vi "main_locate.vi"() -> ()   [LabVIEW 2023]
uses:
  subVis/HologramInfo.ctl
  <vilib>/Math Plots/3D Math Plots/3D Scatter/3D Scatter XCtrl/3D Scatter.xctl
  <vilib>/Math Plots/3D Math Plots/3D Scatter/3D Scatter Datatype/3D Scatter Datatype.lvclass
  HoloPyLib/CCL_parameters.ctl
  subVis/referencesBtns.ctl
  subVis/datas.ctl
  <vilib>/Math Plots/3D Math Plots/3D Scatter/3D Scatter Datatype/Public/Plot Helper (Vector).vi
  subVis/globState.vi
  <vilib>/Python/Open Venv Python Session.vi
  HoloPyLib/holoPyTracks.lvlib
panel:
  out "Status":string
  in  "result tab":enum32{"Holograms", "Localisations", "About..."}(tab)
  out "2D Picture":picture caption="Hologram plane number 152"
  out "3D Scatter":refnum<class "3D Plot Datatype.lvclass">[](xcontrol)
  in  "Tab Control":enum32{"PATH", "PARAMETERS", "ACTIONS"}(tab)=enum."ACTIONS"
  in  "HoloDir":path=path "C:/TRAVAIL/developpement/imagesHolo/1000im_manip3" caption="Holograms directory"
  in  "HoloPath":path=path "C:/TRAVAIL/developpement/imagesHolo/1000im_manip3/100um_40x_int_.7ajmvz4e.000000.bmp" caption="Test hologram path"
  in  "PythonVer":string="3.10" caption="Python version"
  in  "Python/Environnement\npath":path
  in  "Fourier BP filter (pix)":T1={"High pass (0=none)"=15.0, "Low Pass (0=none)"=125.0} {"Low Pass (0=none)" format="%#_6f"}
  in  "CCL parameters":T2={"Threshold ( N x Standard deviation)"=10.0, "Connectivity"=enum."26", "min voxel"=1.0, "max voxel"=0.0} {"max voxel" min=0.0 max=0.0; "min voxel" min=1.0 max=100.0; "Threshold ( N x Standard deviation)" min=1.0 max=100.0}
  in  "Batch thresold":T3(ring)
  in  "Focus":T4={"Type"=enum."SUM_OF_VARIANCE", "Sum size"=15} {"Sum size" min=1 max=100}
  in  "propagation":T5={"distance ini"=0.0, "number of planes"=100, "step"=1e-06} {"step" format="%#_6e"; "distance ini" format="%#_6e"}
  in  "Remove mean Hologram":bool=TRUE
  in  "HoloParam":T6={"wavelength"=6.6e-07, "optical index"=1.33, "Holo size X"=1024, "Holo size Y"=1024, "pixel size"=7e-06, "objective magnification"=40.0} caption="Holo parameters" {"wavelength" format="%#_6e"}
  in  "exitTestMode":bool
  in  "testMode":bool
  in  "CANCEL_BATCH":bool
  in  "EXIT":bool
  in  "BATCH":bool
  in  "Plane number":u16=95 max=200
  in  "Display":T7(ring)
  # "Analyse parameters"
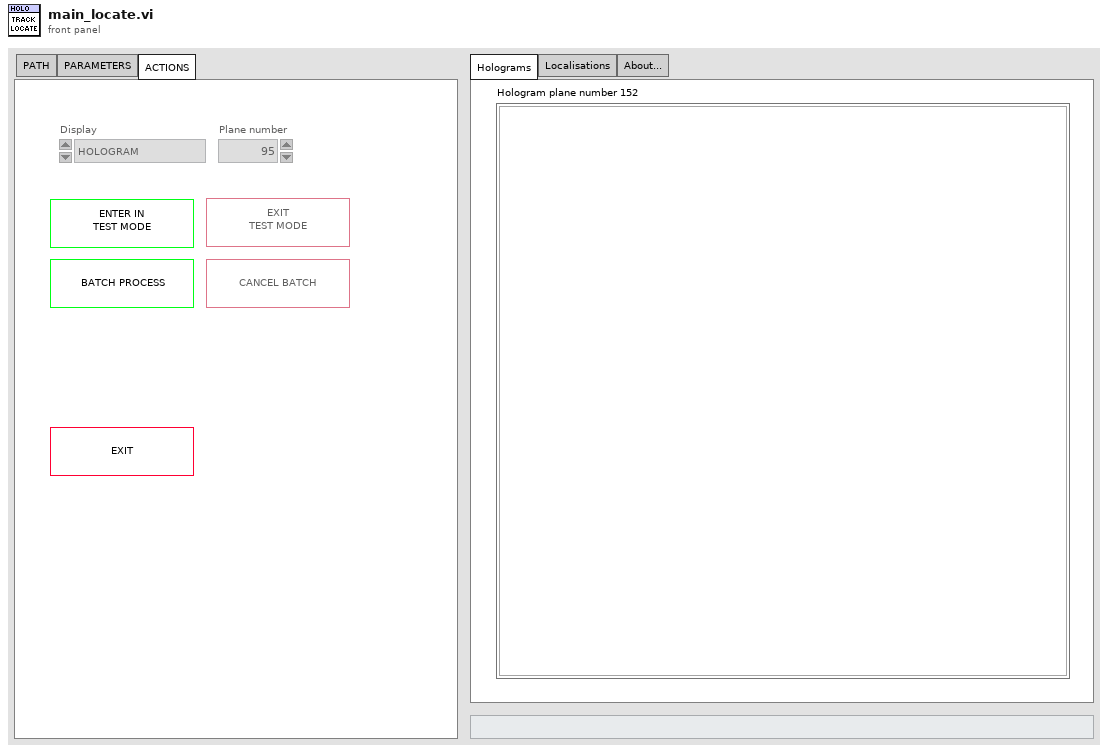
[diagram p1: front panel]
types:
  T1 = cluster{"High pass (0=none)":dbl, "Low Pass (0=none)":dbl}
  T2 = typedef "CCL_parameters.ctl" = cluster{"Threshold ( N x Standard deviation)":dbl, "Connectivity":enum16{"6", "18", "26"}, "min voxel":dbl, "max voxel":dbl}
  T3 = enum16{"compute on 1st hologram", "compute on each hologram"}
  T4 = cluster{"Type":enum16{"SUM_OF_INTENSITY", "SUM_OF_LAPLACIAN", "SUM_OF_VARIANCE", "TENENGRAD"}, "Sum size":i32}
  T5 = cluster{"distance ini":dbl, "number of planes":i32, "step":dbl}
  T6 = typedef "holoPyTracks.lvlib/HologramInfo.ctl" = cluster{"wavelength":sgl, "optical index":sgl, "Holo size X":i32, "Holo size Y":i32, "pixel size":sgl, "objective magnification":sgl}
  T7 = enum16{"HOLOGRAM", "XY PLANE NUMBER....", "XY MAX PLANE", "XY SUM PLANE", "XZ MAX PLANE", "XZ SUM PLANE", "YZ MAX PLANE", "YZ SUM PLANE"}
  T8 = typedef "referencesBtns.ctl" = cluster{"PythonVer":refnum<vi>, "Python/Environnement\npath":refnum<vi>, "HoloPath":refnum<vi>, "HoloDir":refnum<vi>, "Holo parameters":refnum<vi>, "Remove mean Hologram":refnum<vi>, "propagation":refnum<vi>, "Fourier BP filter (pix)":refnum<vi>, "Focus":refnum<vi>, "Batch thresold ":refnum<vi>, "CCL parameters":refnum<vi>, "testMode":refnum<vi>, "exitTestMode":refnum<vi>, "BATCH":refnum<vi>, "CANCEL_BATCH":refnum<vi>, "EXIT":refnum<vi>, "Plane number":refnum<vi>, "Display":refnum<vi>}
  T9 = typedef "param_defaut.ctl" = cluster{"PythonVer":string, "Python/Environnement\npath":path, "HoloPath":path, "HoloDir":path, "HoloParam":T6, "Remove mean Hologram":bool, "propagation":cluster{"distance ini":dbl, "number of planes":i32, "step":dbl}, "Fourier BP filter (pix)":cluster{"High pass (0=none)":dbl, "Low Pass (0=none)":dbl}, "Focus":cluster{"Type":enum16{"SUM_OF_INTENSITY", "SUM_OF_LAPLACIAN", "SUM_OF_VARIANCE", "TENENGRAD"}, "Sum size":i32}, "Batch thresold ":enum16{"compute on 1st hologram", "compute on each hologram"}, "CCL parameters":T2}
  T10 = enum16{"SESSION CLOSED", "WAIT", "TEST WAIT", "TEST IN PROGESS", "BATCH IN PROGRESS"}
  T11 = typedef "datas.ctl" = cluster{"PythonSession":refnum<k35>, "Display":bool, "BinThreshold":sgl, "LIST HOLO BATCH":path[], "Display":sgl[][], "meanHolo":sgl[][], "FEATURES(µm)":sgl[][], "LabelPicture":string, "Status":string, "planeToDisplayFeatures":enum16{"XY", "XZ", "YZ"}, "State":enum16{"SESSION CLOSED", "WAIT", "TEST WAIT", "TEST IN PROGESS", "BATCH IN PROGRESS"}}
  T12 = cluster{"Remove mean Hologram":bool, "Binarisation thresold ":enum16{"compute on 1st hologram", "compute on each hologram"}, "LIST HOLO BATCH":path[], "HoloDir":path}
  T13 = cluster{"Holo parameters":T6, "propagation":cluster{"distance ini":dbl, "number of planes":i32, "step":dbl}, "Fourier BP filter (pix)":cluster{"High pass (0=none)":dbl, "Low Pass (0=none)":dbl}, "Focus":cluster{"Type":enum16{"SUM_OF_INTENSITY", "SUM_OF_LAPLACIAN", "SUM_OF_VARIANCE", "TENENGRAD"}, "Sum size":i32}, "CCL parameters":T2}
  T14 = cluster{"Display":enum16{"HOLOGRAM", "XY PLANE NUMBER....", "XY MAX PLANE", "XY SUM PLANE", "XZ MAX PLANE", "XZ SUM PLANE", "YZ MAX PLANE", "YZ SUM PLANE"}, "Plane number":u16}
  T15 = cluster{"HOLO_array":sgl[][], "FEATURES(µm)":sgl[][], "Features(pix)":sgl[][], "planeToDisplayFeatures":enum16{"XY", "XZ", "YZ"}, "label":string}
  T16 = cluster{"X":i32, "Y":i32, "Z":i32, "XYsize":i32, "ZSize":i32}
  T17 = typedef "eventvkey.ctl" = enum16{"ASCII", "Enter", "Return", "Shift", "Ctrl", "Alt", "Cmd", "Opt", "Caps", "NumLock", "Clear", "Break", "Up", "Down", "Left", "Right", "Insert", "Delete", "Home", "End", "PageUp", "PageDown", "Escape", "Help", "Pause", "ScrollLock", "F1", "F2", "F3", "F4", "F5", "F6", "F7", "F8", "F9", "F10", "F11", "F12", "F13", "F14", "F15", "F16", "F17", "F18", "F19", "F20", "F21", "F22", "F23", "F24", "Play", "VolumeUp", "VolumeDown", "Mute", "Two Byte Char"}
  T18 = cluster{"Display":enum16{"HOLOGRAM", "XY PLANE NUMBER....", "XY MAX PLANE", "XY SUM PLANE", "XZ MAX PLANE", "XZ SUM PLANE", "YZ MAX PLANE", "YZ SUM PLANE"}, u16}
  T19 = cluster{"PythonVer":string, "Python/Environnement\npath":path, "HoloPath":path, "HoloDir":path, "HoloParam":T6, "Remove mean Hologram":bool, "propagation":cluster{"distance ini":dbl, "number of planes":i32, "step":dbl}, "Fourier BP filter (pix)":cluster{"High pass (0=none)":dbl, "Low Pass (0=none)":dbl}, "Focus":cluster{"Type":enum16{"SUM_OF_INTENSITY", "SUM_OF_LAPLACIAN", "SUM_OF_VARIANCE", "TENENGRAD"}, "Sum size":i32}, "Batch thresold ":enum16{"compute on 1st hologram", "compute on each hologram"}, "CCL parameters":T2}
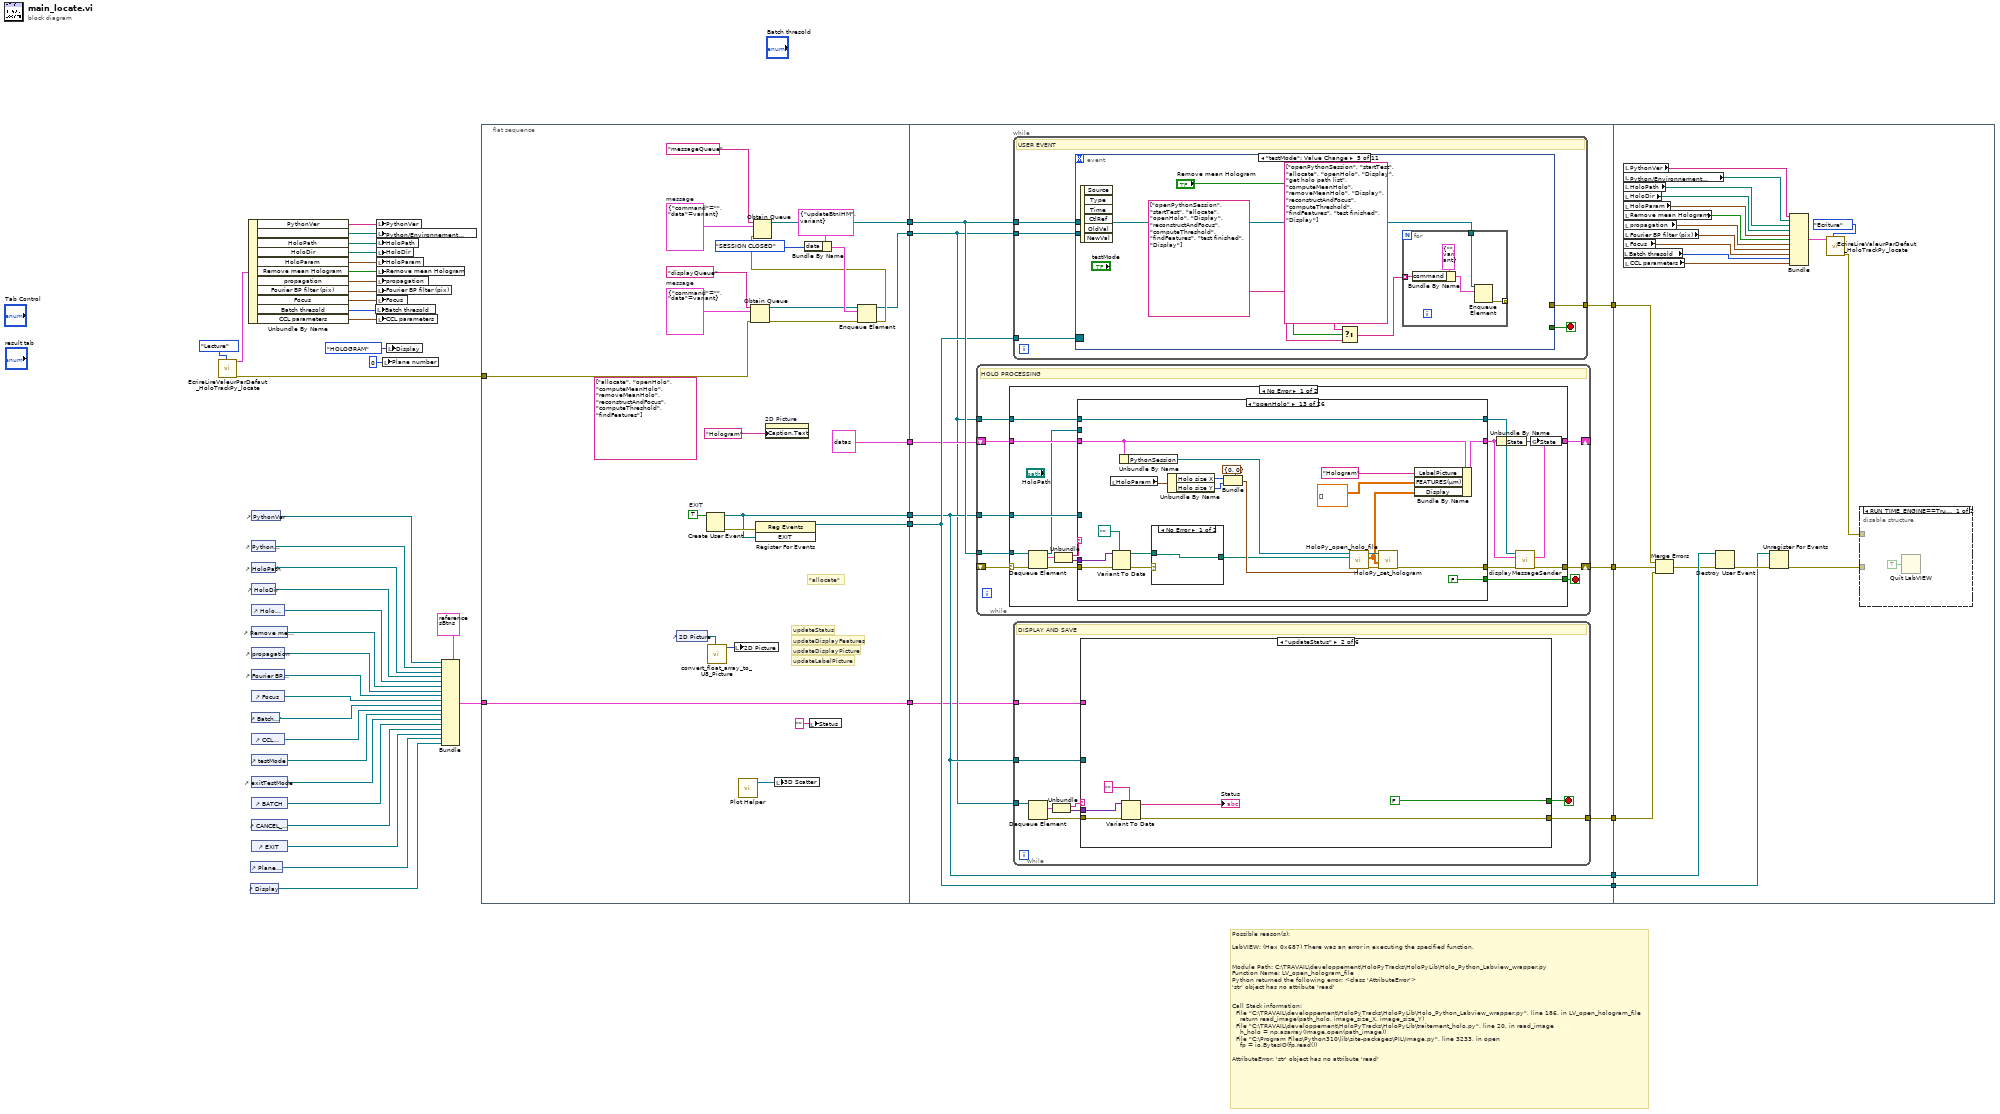
[diagram p0: block diagram]
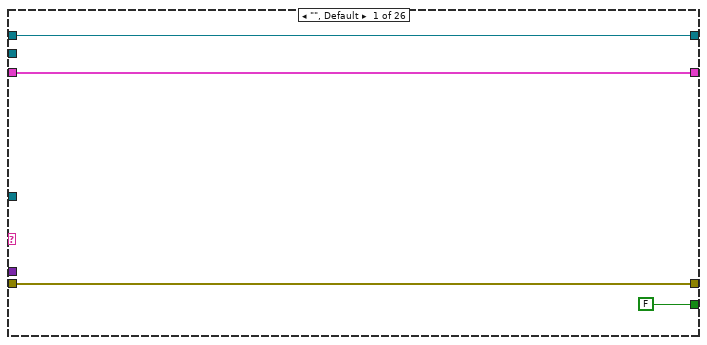
[diagram p2: hidden frame]
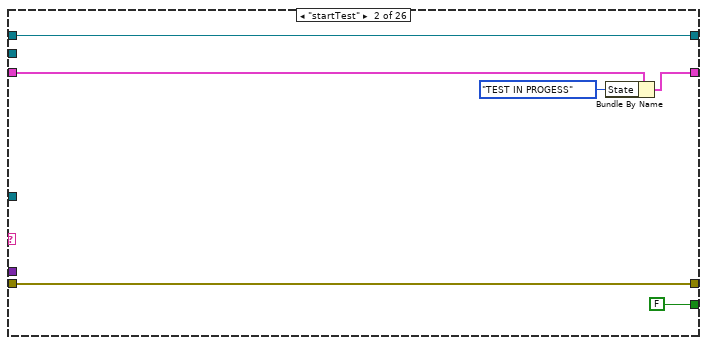
[diagram p3: hidden frame]
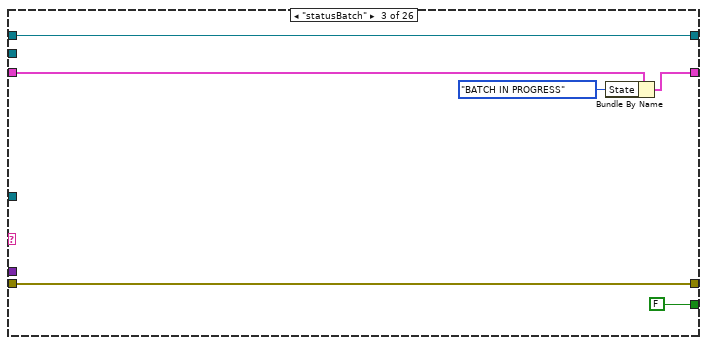
[diagram p4: hidden frame]
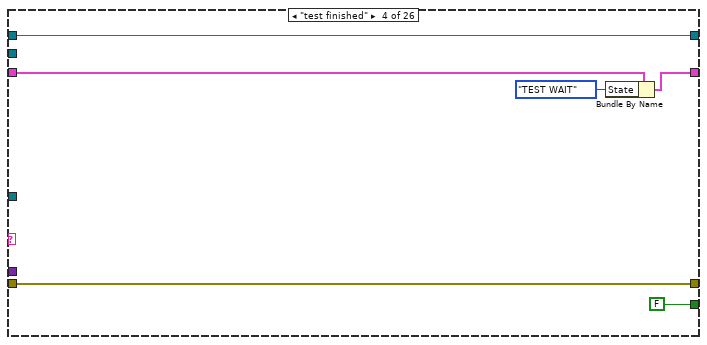
[diagram p5: hidden frame]
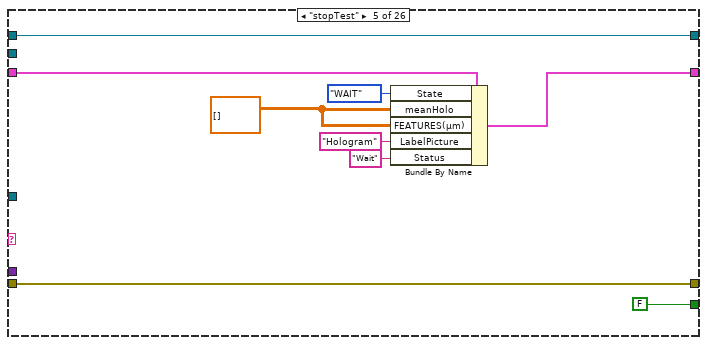
[diagram p6: hidden frame]
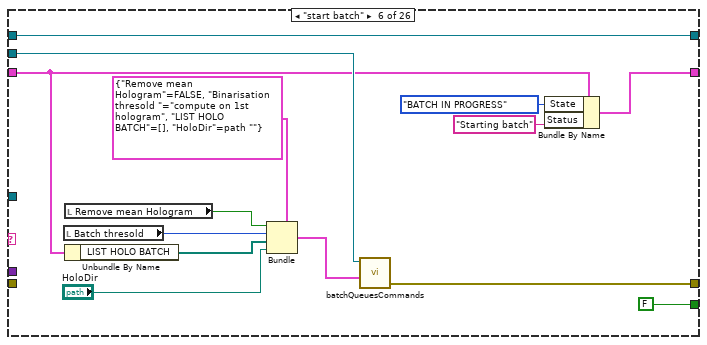
[diagram p7: hidden frame]
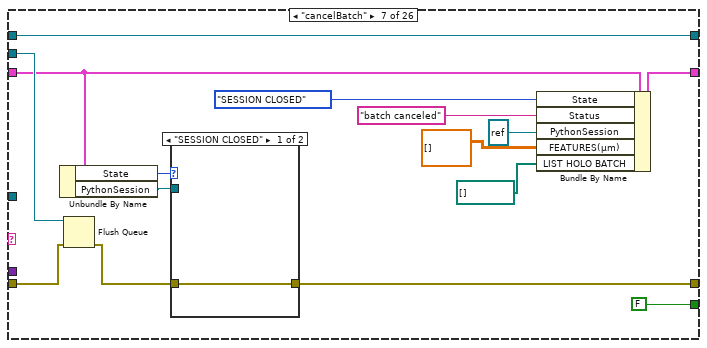
[diagram p8: hidden frame]
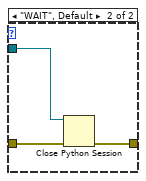
[diagram p9: hidden frame]
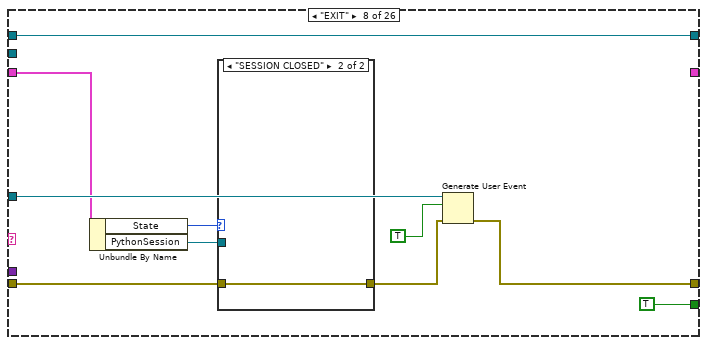
[diagram p10: hidden frame]
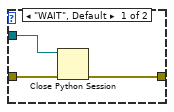
[diagram p11: hidden frame]
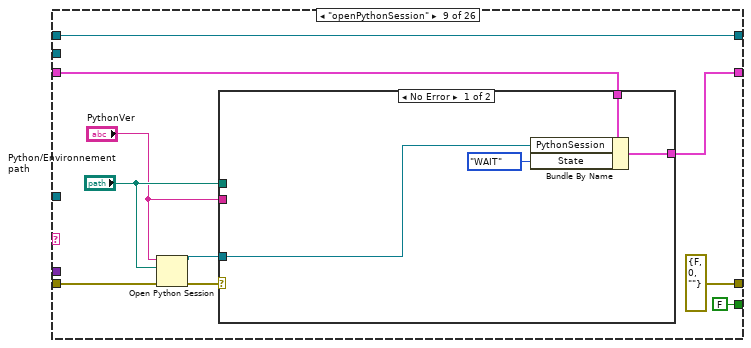
[diagram p12: hidden frame]
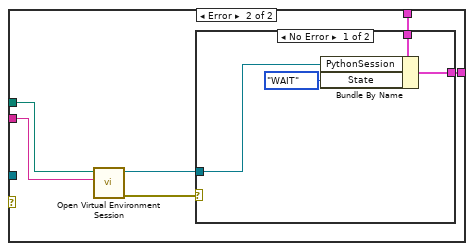
[diagram p13: hidden frame]
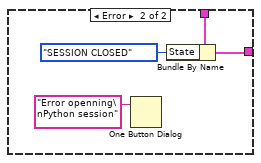
[diagram p14: hidden frame]
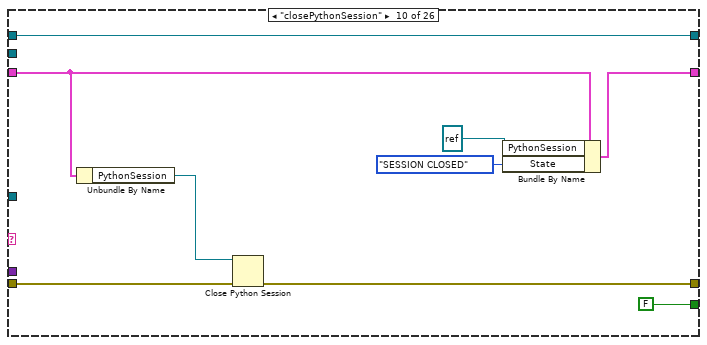
[diagram p15: hidden frame]
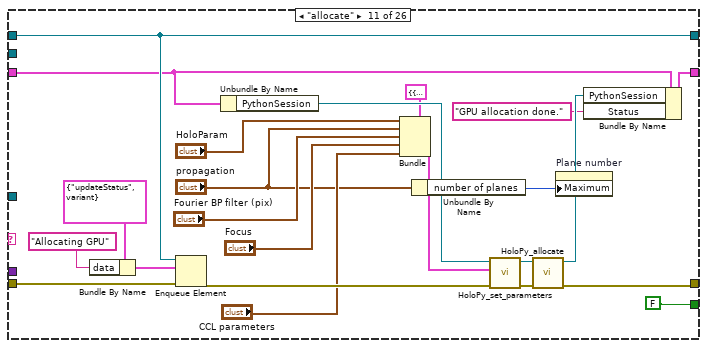
[diagram p16: hidden frame]
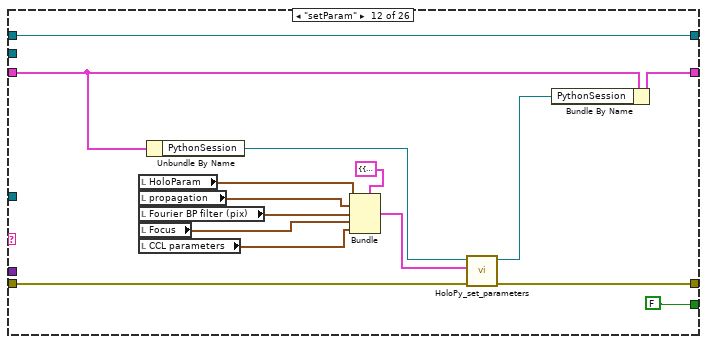
[diagram p17: hidden frame]
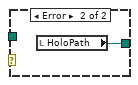
[diagram p18: hidden frame]
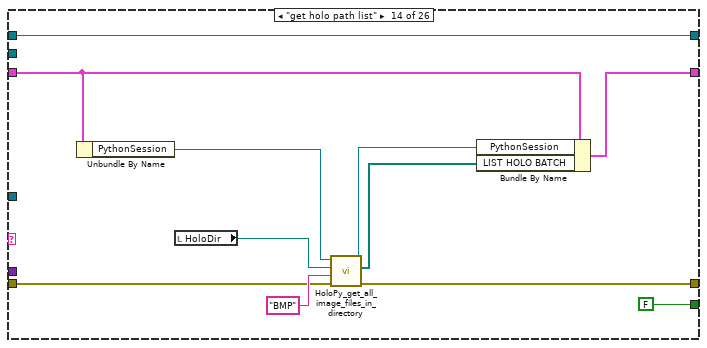
[diagram p19: hidden frame]
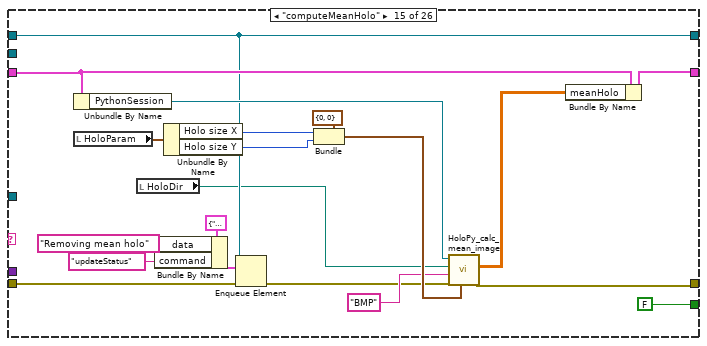
[diagram p20: hidden frame]
diagram:
  # "Possible reason(s):\n\nLabVIEW: (Hex 0x687) There was an error in executing the specified function.\n\n\nModule Path: C:\\TRAVAIL\\developpement\\HoloPyTracks\\HoloPyLib\\Holo_Python_Labview_wrapper.py\nFunction Name: LV_open_hologram_file\nPython returned the following error: <class 'AttributeError'>\n'str' object has no attribute 'read'\n\n\nCall Stack information:\n  File \"C:\\TRAVAIL\\developpement\\HoloPyTracks\\HoloPyLib\\Holo_Python_Labview_wrapper.py\", line 186, in LV_open_hologram_file\n    return read_image(path_holo, image_size_X, image_size_Y)\n  File \"C:\\TRAVAIL\\developpement\\HoloPyTracks\\HoloPyLib\\traitement_holo.py\", line 20, in read_image\n    h_holo = np.asarray(Image.open(path_image))\n  File \"C:\\Program Files\\Python310\\lib\\site-packages\\PIL\\Image.py\", line 3233, in open\n    fp = io.BytesIO(fp.read())\n\nAttributeError: 'str' object has no attribute 'read'"
  n1 = call "EcrireLireValeurParDefaut_HoloTrackPy_locate.vi"("Lecture/Ecriture"=enum32{"Lecture", "Ecriture"}."Lecture") -> ("error out"=w31:errorcluster, "ParamOUT"=w33:T9)  [unwired: 7 in, 2 out]
  n2 = Unbundle By Name(w33) -> ("PythonVer"=w18:string, "Python/Environnement\npath"=w17:path, "HoloPath"=w16:path, "HoloDir"=w15:path, "HoloParam"=w14:T6, "Remove mean Hologram"=w13:bool, "propagation"=w12:T5, "Fourier BP filter (pix)"=w11:T1, "Focus"=w10:T4, "Batch thresold"=w9:T3, "CCL parameters"=w8:T2)
  n3 = control-ref of="Plane number"() -> (w7:refnum<vi>)
  n4 = control-ref of="Display"() -> (w1:refnum<vi>)
  n5 = control-ref of="PythonVer"() -> (w29:refnum<vi>)
  n6 = control-ref of="Python/Environnement\npath"() -> (w30:refnum<vi>)
  n7 = control-ref of="HoloPath"() -> (w38:refnum<vi>)
  n8 = control-ref of="HoloDir"() -> (w37:refnum<vi>)
  n9 = control-ref of="Holo parameters"() -> (w36:refnum<vi>)
  n10 = control-ref of="Remove mean Hologram"() -> (w28:refnum<vi>)
  n11 = control-ref of="propagation"() -> (w27:refnum<vi>)
  n12 = control-ref of="Fourier BP filter (pix)"() -> (w26:refnum<vi>)
  n13 = control-ref of="Focus"() -> (w25:refnum<vi>)
  n14 = control-ref of="Batch thresold"() -> (w24:refnum<vi>)
  n15 = control-ref of="CCL parameters"() -> (w23:refnum<vi>)
  n16 = control-ref of="testMode"() -> (w22:refnum<vi>)
  n17 = control-ref of="exitTestMode"() -> (w21:refnum<vi>)
  n18 = control-ref of="BATCH"() -> (w20:refnum<vi>)
  n19 = control-ref of="CANCEL_BATCH"() -> (w19:refnum<vi>)
  n20 = control-ref of="EXIT"() -> (w35:refnum<vi>)
  n21 = local write "Batch thresold"(w9) -> ()
  n22 = local write "PythonVer"(w18) -> ()
  n23 = local write "Python/Environnement\npath"(w17) -> ()
  n24 = local write "HoloPath"(w16) -> ()
  n25 = local write "HoloDir"(w15) -> ()
  n26 = local write "HoloParam"(w14) -> ()
  n27 = local write "Remove mean Hologram"(w13) -> ()
  n28 = local write "propagation"(w12) -> ()
  n29 = local write "Fourier BP filter (pix)"(w11) -> ()
  n30 = local write "Focus"(w10) -> ()
  n31 = local write "CCL parameters"(w8) -> ()
  n32 = local write "Plane number"(u16 0 ("Plane number")) -> ()
  n33 = local write "Display"(T7."HOLOGRAM" ("Display")) -> ()
  n34 = Bundle(cluster=T8 {"PythonVer"=refnum, "Python/Environnement\npath"=refnum, "HoloPath"=refnum, "HoloDir"=refnum, "Holo parameters"=refnum, "Remove mean Hologram"=refnum, "propagation"=refnum, "Fourier BP filter (pix)"=refnum, "Focus"=refnum, "Batch thresold "=refnum, "CCL parameters"=refnum, "testMode"=refnum, "exitTestMode"=refnum, "BATCH"=refnum, "CANCEL_BATCH"=refnum, "EXIT"=refnum, "Plane number"=refnum, "Display"=refnum} ("output cluster"), "PythonVer"=w29, "Python/Environnement\npath"=w30, "HoloPath"=w38, "HoloDir"=w37, "Holo parameters"=w36, "Remove mean Hologram"=w28, "propagation"=w27, "Fourier BP filter (pix)"=w26, "Focus"=w25, "Batch thresold"=w24, "CCL parameters"=w23, "testMode"=w22, "exitTestMode"=w21, "BATCH"=w20, "CANCEL_BATCH"=w19, "EXIT"=w35, "Plane number"=w7, "Display"=w1) -> (w5:T8)
  n35 = flat-sequence {
    tunnel: [w67] -> w47
    tunnel: [w66] -> w46
    tunnel: [w49] -> w45
    tunnel: [T11 {"PythonSession"=refnum, "Display"=FALSE, "BinThreshold"=0.0, "LIST HOLO BATCH"=[], "Display"=[], "meanHolo"=[], "FEATURES(µm)"=[], "LabelPicture"="", "Status"="", "planeToDisplayFeatures"=enum."XY", "State"=enum."SESSION CLOSED"}] -> w44
    tunnel: [w57] -> w34
    tunnel: w5 -> [w57]
    tunnel: w31 -> [w56]
    tunnel: [w55] -> w4
    tunnel: w47 -> [w77]
    tunnel: w46 -> [w79]
    tunnel: w45 -> [w75]
    tunnel: w44 -> [w76]
    tunnel: [w79] -> w43
    tunnel: [w77] -> w42
    tunnel: [w78] -> w41
    tunnel: [w74] -> w40
    tunnel: [w73] -> w39
    tunnel: w34 -> [w72]
    tunnel: w4 -> [w80]
    tunnel: w43 -> [w858]
    tunnel: w42 -> [w857]
    tunnel: w41 -> [w854]
    tunnel: w40 -> [w856]
    tunnel: w39 -> [w855]
    frame #0 {
      (unwired) string[] ["allocate", "openHolo", "computeMeanHolo", "removeMeanHolo", "reconstructAndFocus", "computeThreshold", "findFeatures"]
      w65 = cluster{"command":string, "data":variant} {"command"="", "data"=variant}  # message
      w69 = TRUE  # EXIT
      w70 = cluster{"command":string, "data":variant} {"command"="", "data"=variant}  # message
      # "\"allocate\""
      # "updateDisplayFeatures"
      # "updateLabelPicture"
      # "updateDisplayPicture"
      # "updateStatus"
      n36 = control-ref of="2D Picture"() -> (w62:refnum<vi>)
      n37 = Create User Event(user event datatype=w69) -> (user event=w67:refnum<user-event>, error out=w68:errorcluster)  [unwired: 1 in]
      n38 = call "convert_float_array_to_U8_Picture.vi"("Pict Refnum"=w62) -> ("new picture"=w61:picture)  [unwired: 9 in, 1 out]
      n39 = local write "2D Picture"(w61) -> ()
      n40 = call-poly <vilib>:"Plot Helper.vi"() -> ("3D Plot lvclass Array out"=w58:refnum<class "3D Plot Datatype.lvclass">[])  [unwired: 6 in, 5 out]
      n41 = Obtain Queue(name (unnamed)="displayQueue", element data type=w65, error in (no error)=w56) -> (queue out=w52:refnum<queue>, error out=w51:errorcluster)  [unwired: 2 in, 1 out]
      n42 = register-events(error in=w68, w67) -> (reference out=w66:refnum<event-registration>)  [unwired: 1 in, 1 out]
      n43 = property on="2D Picture" class="Pict"("Caption.Text"="Hologram" ("Label.Text")) -> ()  [unwired: 2 in, 2 out]
      n44 = local write "3D Scatter"(w58) -> ()
      n45 = Bundle By Name(cluster=cluster{"command":string, "data":variant} {"command"="updateBtnIHM", "data"=variant} ("element"), "data"=T10."SESSION CLOSED" ("State")) -> (w53:cluster{"command":string, "data":variant})
      n46 = local write "Status"("" ("Status")) -> ()
      n47 = Enqueue Element(queue=w52, element=w53, error in (no error)=w51) -> (queue out=w49:refnum<queue>, error out=w50:errorcluster)  [unwired: 1 in, 1 out]
      n48 = Obtain Queue(name (unnamed)="messageQueue", element data type=w70, error in (no error)=w50) -> (queue out=w55:refnum<queue>)  [unwired: 2 in, 2 out]
    }
    frame #1 {
      n49 = while {
        tunnel: w80 -> [w88]
        tunnel: w77 -> [w86]
        shift-right: [w84] -> _
        shift-left: w76 -> [w85]
        tunnel: w75 -> [w83]
        shift-right: [w82] -> w73
        shift-left: _ -> [w81]
        stop <- w87 stop-if-true
        # "HOLO PROCESSING"
        n50 = case shown="No Error" w81 {
          selector: w81 -> [w95 w653]
          tunnel: w88 -> [w105 w654]
          tunnel: [w100 FALSE] -> w87
          tunnel: w86 -> [w99 _]
          tunnel: w85 -> [w98 w649]
          tunnel: [w91 w649] -> w84
          tunnel: w83 -> [w97 _]
          tunnel: [w93 errorcluster {"status"=FALSE, "code"=0, "source"=""} ("error out")] -> w82
          frame No Error {
            n51 = Dequeue Element(queue=w105, error in (no error)=w95) -> (queue out=w96:refnum<queue>, element=w103:cluster{"command":string, "data":variant}, error out=w104:errorcluster)  [unwired: 1 in, 1 out]
            n52 = Unbundle(w103) -> ("command"=w102:string, "data"=w101:variant)
            n53 = case shown="\"openHolo\"" w102 {
              tunnel: w104 -> [w107 w111 w117 w123 w129 _ w161 w175 w191 w216 w239 w253 w262 w285 w301 w316 w335 w344 w368 w402 w575 w587 w610 w626 w630 w647]
              tunnel: w101 -> [_ _ _ _ _ _ _ _ _ _ _ _ w261 _ _ _ _ _ w367 w401 _ w586 w609 w625 _ w646]
              tunnel: [FALSE FALSE FALSE FALSE FALSE FALSE FALSE TRUE FALSE FALSE FALSE FALSE FALSE FALSE FALSE FALSE FALSE FALSE FALSE FALSE FALSE FALSE FALSE FALSE FALSE FALSE] -> w100
              tunnel: w99 -> [_ _ _ _ _ _ _ w178 _ _ _ _ _ _ _ _ _ _ _ _ _ _ _ _ _ _]
              tunnel: w98 -> [w108 w113 w119 w125 w134 w144 w155 w170 w188 w215 w236 w252 w276 w291 w308 w322 w332 w342 w363 w405 w579 w593 w605 w624 w636 w640]
              tunnel: [w108 w112 w118 w124 w133 w146 w164 _ w187 w217 w242 w257 w275 w292 w307 w321 w331 w341 w362 w405 w578 w592 w604 w623 w635 w640] -> w90
              tunnel: w97 -> [w106 w114 w120 w126 w135 w147 w160 w171 w192 w219 w238 w256 w272 w286 w299 w320 w333 w339 w364 w404 w580 w594 w603 w622 w634 w638]
              tunnel: [w107 w111 w117 w123 w129 w148 w153 w172 errorcluster {"status"=FALSE, "code"=0, "source"=""} ("error out") w213 w234 w255 w270 w288 w300 w319 w330 w343 w351 w406 w574 w589 w598 w614 w633 w643] -> w92
              tunnel: w96 -> [_ _ _ _ _ w149 w162 _ _ _ _ _ _ _ _ _ _ _ _ _ _ _ _ _ _ _]
              tunnel: [w106 w114 w120 w126 w135 w147 w160 w171 w192 w219 w238 w256 w272 w286 w299 w320 w333 w339 w364 w404 w580 w594 w603 w622 w634 w638] -> w94
              frame "", Default {
              }
              frame "startTest" {
                n54 = Bundle By Name(cluster=w113, "State"=T10."TEST IN PROGESS") -> (w112:T11)
              }
              frame "statusBatch" {
                n55 = Bundle By Name(cluster=w119, "State"=T10."BATCH IN PROGRESS") -> (w118:T11)
              }
              frame "test finished" {
                n56 = Bundle By Name(cluster=w125, "State"=T10."TEST WAIT") -> (w124:T11)
              }
              frame "stopTest" {
                w130 = sgl[][] [] ("meanHolo")
                n57 = Bundle By Name(cluster=w134, "State"=T10."WAIT", "meanHolo"=w130, "FEATURES(µm)"=w130, "LabelPicture"="Hologram", "Status"="Wait") -> (w133:T11)
              }
              frame "start batch" {
                n58 = local read "Batch thresold"() -> (w142:T3)
                n59 = local read "Remove mean Hologram"() -> (w143:bool)
                n60 = Unbundle By Name(w144) -> ("LIST HOLO BATCH"=w141:path[])
                n61 = Bundle(cluster=T12 {"Remove mean Hologram"=FALSE, "Binarisation thresold "=enum."compute on 1st hologram", "LIST HOLO BATCH"=[], "HoloDir"=path ""} ("Batch parameters"), "Remove mean Hologram"=w143, "Binarisation thresold"=w142, "LIST HOLO BATCH"=w141, "HoloDir"="HoloDir") -> (w140:T12)
                n62 = call "batchQueuesCommands.vi"("Batch parameters"=w140, "QueueMessages"=w149) -> ("error out"=w148:errorcluster)  [unwired: 9 in]
                n63 = Bundle By Name(cluster=w144, "State"=T10."BATCH IN PROGRESS", "Status"="Starting batch") -> (w146:T11)
              }
              frame "cancelBatch" {
                n64 = Unbundle By Name(w155) -> ("State"=w154:T10, "PythonSession"=w151:refnum<k35>)
                n65 = Flush Queue(queue=w162, error in (no error)=w161) -> (error out=w152:errorcluster)  [unwired: 2 out]
                n66 = case shown="\"SESSION CLOSED\"" w154 {
                  tunnel: [w166 w167] -> w153
                  tunnel: w152 -> [w166 w169]
                  tunnel: w151 -> [_ w168]
                  frame "SESSION CLOSED" {
                  }
                  frame "WAIT", Default {
                    n67 = Close Python Session(session in=w168, error in=w169) -> (11:w167:errorcluster)
                  }
                }
                n68 = Bundle By Name(cluster=w155, "State"=T10."SESSION CLOSED", "Status"="batch canceled" ("command"), "PythonSession"=refnum<k35> refnum, "FEATURES(µm)"=sgl[][] [] ("Holo"), "LIST HOLO BATCH"=path[] []) -> (w164:T11)
              }
              frame "EXIT" {
                n69 = Unbundle By Name(w170) -> ("State"=w176:T10, "PythonSession"=w174:refnum<k35>)
                n70 = case shown="\"SESSION CLOSED\"" w176 {
                  tunnel: w175 -> [w182 w183]
                  tunnel: w174 -> [w181 _]
                  tunnel: [w180 w183] -> w173
                  frame "WAIT", Default {
                    n71 = Close Python Session(session in=w181, error in=w182) -> (11:w180:errorcluster)
                  }
                  frame "SESSION CLOSED" {
                  }
                }
                n72 = Generate User Event(user event=w178, event data cluster=TRUE ("event data"), error in=w173) -> (error out=w172:errorcluster)  [unwired: 1 in, 1 out]
              }
              frame "openPythonSession" {
                n73 = Open Python Session(python version="PythonVer", python path="Python/Environnement\npath", 3:w191) -> (session out=w185:refnum<k35>, error out=w190:errorcluster)
                n74 = case shown="No Error" w190 {
                  tunnel: "Python/Environnement\npath" -> [_ w203]
                  tunnel: "PythonVer" -> [_ w202]
                  tunnel: w188 -> [w197 w200]
                  tunnel: [w196 w199] -> w187
                  tunnel: w185 -> [w195 _]
                  frame No Error {
                    n75 = Bundle By Name(cluster=w197, "PythonSession"=w195, "State"=T10."WAIT") -> (w196:T11)
                  }
                  frame Error {
                    n76 = call-poly <vilib>:"Open Virtual Environment Session.vi"("Python version"=w202, "Env path"=w203) -> ("error out"=w201:errorcluster, "session out"=w198:refnum<k35>)  [unwired: 8 in]
                    n77 = case shown="No Error" w201 {
                      tunnel: w200 -> [w207 w210]
                      tunnel: [w206 w209] -> w199
                      tunnel: w198 -> [w205 _]
                      frame No Error {
                        n78 = Bundle By Name(cluster=w207, "PythonSession"=w205, "State"=T10."WAIT") -> (w206:T11)
                      }
                      frame Error {
                        n79 = One Button Dialog(message="Error openning\nPython session") -> ()  [unwired: 1 in, 1 out]
                        n80 = Bundle By Name(cluster=w210, "State"=T10."SESSION CLOSED") -> (w209:T11)
                      }
                    }
                  }
                }
              }
              frame "closePythonSession" {
                n81 = Unbundle By Name(w215) -> ("PythonSession"=w214:refnum<k35>)
                n82 = Close Python Session(session in=w214, error in=w216) -> (11:w213:errorcluster)
                n83 = Bundle By Name(cluster=w215, "PythonSession"=refnum<k35> refnum, "State"=T10."SESSION CLOSED") -> (w217:T11)
              }
              frame "allocate" {
                n84 = Bundle By Name(cluster=cluster{"command":string, "data":variant} {"command"="updateStatus", "data"=variant} ("element"), "data"="Allocating GPU" ("command")) -> (w237:cluster{"command":string, "data":variant})
                n85 = Enqueue Element(queue=w238, element=w237, error in (no error)=w239) -> (error out=w232:errorcluster)  [unwired: 1 in, 2 out]
                n86 = Unbundle By Name(w236) -> ("PythonSession"=w230:refnum<k35>)
                n87 = Bundle(cluster=T13 {"Holo parameters"={"wavelength"=0.0, "optical index"=0.0, "Holo size X"=0, "Holo size Y"=0, "pixel size"=0.0, "objective magnification"=0.0}, "propagation"={"distance ini"=0.0, "number of planes"=0, "step"=0.0}, "Fourier BP filter (pix)"={"High pass (0=none)"=0.0, "Low Pass (0=none)"=0.0}, "Focus"={"Type"=enum."SUM_OF_INTENSITY", "Sum size"=0}, "CCL parameters"={"Threshold ( N x Standard deviation)"=0.0, "Connectivity"=enum."6", "min voxel"=0.0, "max voxel"=0.0}} ("ParametersIN"), "Holo parameters"="HoloParam", "propagation"="propagation", "Fourier BP filter (pix)"="Fourier BP filter (pix)", "Focus"="Focus", "CCL parameters"="CCL parameters") -> (w228:T13)
                n88 = Unbundle By Name("propagation") -> ("number of planes"=w221:i32)
                n89 = call "HoloPy_set_parameters.vi"("error in (no error)"=w232, "ParametersIN"=w228, "session in"=w230) -> ("error out"=w231:errorcluster, "Refnum out"=w229:refnum<k35>)  [unwired: 6 in, 1 out]
                n90 = call "HoloPy_allocate.vi"("error in (no error)"=w231, "session in"=w229) -> ("error out"=w234:errorcluster, "Refnum out"=w235:refnum<k35>)  [unwired: 7 in, 1 out]
                n91 = property on="Plane number" class="DigNum (strict)"("Maximum"=w221) -> ()  [unwired: 2 in, 2 out]
                n92 = Bundle By Name(cluster=w236, "PythonSession"=w235, "Status"="GPU allocation done." ("command")) -> (w242:T11)
              }
              frame "setParam" {
                n93 = local read "HoloParam"() -> (w249:T6)
                n94 = local read "propagation"() -> (w248:T5)
                n95 = local read "Fourier BP filter (pix)"() -> (w247:T1)
                n96 = local read "Focus"() -> (w246:T4)
                n97 = local read "CCL parameters"() -> (w245:T2)
                n98 = Unbundle By Name(w252) -> ("PythonSession"=w251:refnum<k35>)
                n99 = Bundle(cluster=T13 {"Holo parameters"={"wavelength"=0.0, "optical index"=0.0, "Holo size X"=0, "Holo size Y"=0, "pixel size"=0.0, "objective magnification"=0.0}, "propagation"={"distance ini"=0.0, "number of planes"=0, "step"=0.0}, "Fourier BP filter (pix)"={"High pass (0=none)"=0.0, "Low Pass (0=none)"=0.0}, "Focus"={"Type"=enum."SUM_OF_INTENSITY", "Sum size"=0}, "CCL parameters"={"Threshold ( N x Standard deviation)"=0.0, "Connectivity"=enum."6", "min voxel"=0.0, "max voxel"=0.0}} ("ParametersIN"), "Holo parameters"=w249, "propagation"=w248, "Fourier BP filter (pix)"=w247, "Focus"=w246, "CCL parameters"=w245) -> (w250:T13)
                n100 = call "HoloPy_set_parameters.vi"("error in (no error)"=w253, "ParametersIN"=w250, "session in"=w251) -> ("error out"=w255:errorcluster, "Refnum out"=w254:refnum<k35>)  [unwired: 6 in, 1 out]
                n101 = Bundle By Name(cluster=w252, "PythonSession"=w254) -> (w257:T11)
              }
              frame "openHolo" {
                n102 = local read "HoloParam"() -> (w268:T6)
                n103 = Variant To Data(error in=w262, type=path "" ("HoloPath"), Variant=w261) -> (data=w263:path, error out=w264:errorcluster)
                n104 = Unbundle By Name(w276) -> ("PythonSession"=w279:refnum<k35>)
                n105 = case shown="No Error" w264 {
                  tunnel: w263 -> [w281 _]
                  tunnel: [w281 w282] -> w259
                  frame No Error {
                  }
                  frame Error {
                    n106 = local read "HoloPath"() -> (w282:path)
                  }
                }
                n107 = Unbundle By Name(w268) -> ("Holo size X"=w267:i32, "Holo size Y"=w266:i32)
                n108 = Bundle(cluster=cluster{"image_size_X":i32, "image_size_Y":i32} {"image_size_X"=0, "image_size_Y"=0} ("imageSize"), "image_size_X"=w267, "image_size_Y"=w266) -> (w277:cluster{"image_size_X":i32, "image_size_Y":i32})
                n109 = call "HoloPy_open_holo_file.vi"("imageSize"=w277, "image path"=w259, "Refnum in"=w279) -> ("error out"=w274:errorcluster, "Array"=w265:sgl[][], "Refnum out"=w273:refnum<k35>)  [unwired: 6 in]
                n110 = call "HoloPy_set_hologram.vi"("error in (no error)"=w274, "HOLO_array"=w265, "Refnum in"=w273) -> ("error out"=w270:errorcluster)  [unwired: 6 in, 2 out]
                n111 = Bundle By Name(cluster=w276, "LabelPicture"="Hologram" ("Label.Text"), "FEATURES(µm)"=sgl[][] [], "Display"=w265) -> (w275:T11)
              }
              frame "get holo path list" {
                n112 = Unbundle By Name(w291) -> ("PythonSession"=w290:refnum<k35>)
                n113 = local read "HoloDir"() -> (w284:path)
                n114 = call "HoloPy_get_all_image_files_in_directory.vi"("error in (no error)"=w285, "file_extension"="BMP", "holo directory"=w284, "Refnum in"=w290) -> ("error out"=w288:errorcluster, "path"=w289:path[], "Refnum out"=w283:refnum<k35>)  [unwired: 5 in]
                n115 = Bundle By Name(cluster=w291, "PythonSession"=w283, "LIST HOLO BATCH"=w289) -> (w292:T11)
              }
              frame "computeMeanHolo" {
                n116 = Unbundle By Name(w308) -> ("PythonSession"=w310:refnum<k35>)
                n117 = local read "HoloParam"() -> (w297:T6)
                n118 = local read "HoloDir"() -> (w294:path)
                n119 = Bundle By Name(cluster=cluster{"command":string, "data":variant} {"command"="", "data"=variant} ("element"), "data"="Removing mean holo" ("command"), "command"="updateStatus") -> (w303:cluster{"command":string, "data":variant})
                n120 = Unbundle By Name(w297) -> ("Holo size X"=w296:i32, "Holo size Y"=w295:i32)
                n121 = Enqueue Element(queue=w299, element=w303, error in (no error)=w301) -> (error out=w298:errorcluster)  [unwired: 1 in, 2 out]
                n122 = Bundle(cluster=cluster{"image_size_X":i32, "image_size_Y":i32} {"image_size_X"=0, "image_size_Y"=0} ("imageSize"), "image_size_X"=w296, "image_size_Y"=w295) -> (w311:cluster{"image_size_X":i32, "image_size_Y":i32})
                n123 = call "HoloPy_calc_mean_image.vi"("imageSize"=w311, "error in (no error)"=w298, "imageFileExtension"="BMP", "directory path"=w294, "Refnum in"=w310) -> ("error out"=w300:errorcluster, "Array"=w306:sgl[][])  [unwired: 4 in, 1 out]
                n124 = Bundle By Name(cluster=w308, "meanHolo"=w306) -> (w307:T11)
              }
              frame "removeMeanHolo" {
                n125 = Unbundle By Name(w322) -> ("PythonSession"=w324:refnum<k35>, "meanHolo"=w323:sgl[][])
                n126 = call "HoloPy_get_hologram.vi"("error in (no error)"=w316, "Refnum in"=w324) -> ("error out"=w326:errorcluster, "HOLO_array"=w327:sgl[][], "Refnum out"=w325:refnum<k35>)  [unwired: 7 in]
                n127 = Divide(x=w327, y=w323) -> (x/y=w314:sgl[][])
                n128 = call "HoloPy_set_hologram.vi"("error in (no error)"=w326, "HOLO_array"=w314, "Refnum in"=w325) -> ("error out"=w319:errorcluster, "Refnum out"=w315:refnum<k35>)  [unwired: 6 in, 1 out]
                n129 = Bundle By Name(cluster=w322, "PythonSession"=w315, "LabelPicture"="Hologram", "planeToDisplayFeatures"=enum16{"XY", "XZ", "YZ"}."XY", "Display"=w314) -> (w321:T11)
              }
              frame "reconstructAndFocus" {
                n130 = Unbundle By Name(w332) -> ("PythonSession"=w334:refnum<k35>)
                n131 = call "HoloPy_volume_and_focus.vi"("error in (no error)"=w335, "Refnum in"=w334) -> ("error out"=w330:errorcluster, "Refnum out"=w329:refnum<k35>)  [unwired: 7 in, 1 out]
                n132 = Bundle By Name(cluster=w332, "PythonSession"=w329) -> (w331:T11)
              }
              frame "computeThreshold" {
                n133 = local read "CCL parameters"() -> (w338:T2)
                n134 = Unbundle By Name(w342) -> ("PythonSession"=w349:refnum<k35>)
                n135 = Unbundle By Name(w338) -> ("Threshold ( N x Standard deviation)"=w337:dbl)
                n136 = call "HoloPy_get_mean_std_var_volume.vi"("error in (no error)"=w344, "Refnum in"=w349) -> ("error out"=w343:errorcluster, "data volume"=w348:cluster{"mean":dbl, "std var":dbl})  [unwired: 7 in, 1 out]
                n137 = Unbundle By Name(w348) -> ("mean"=w345:dbl, "std var"=w347:dbl)
                n138 = Multiply(x=w337, y=w347) -> (x*y=w346:dbl)
                n139 = Add(x=w345, y=w346) -> (x+y=w340:dbl)
                n140 = Bundle By Name(cluster=w342, "BinThreshold"=w340) -> (w341:T11)
              }
              frame "findFeatures" {
                n141 = Unbundle By Name(w363) -> ("LIST HOLO BATCH"=w360:path[], "PythonSession"=w365:refnum<k35>, "BinThreshold"=w366:sgl)
                n142 = Variant To Data(error in=w368, type=cluster{"imageNumber":u32, "Display":bool} {"imageNumber"=0, "Display"=TRUE}, Variant=w367) -> (data=w355:cluster{"imageNumber":u32, "Display":bool}, error out=w356:errorcluster)
                n143 = case shown="Error .." w356 {
                  tunnel: w355 -> [w372 _]
                  tunnel: [w371 u32 0 ("imageNumber")] -> w354
                  tunnel: [w370 TRUE ("Display")] -> w353
                  frame No Error {
                    n144 = Unbundle(w372) -> ("imageNumber"=w371:u32, "Display"=w370:bool)
                  }
                  frame Error {
                  }
                }
                n145 = Array Size(array=w360) -> (size(s)=w357:i32)
                n146 = Equal To 0?(x=w354) -> (x = 0?=w359:bool)
                n147 = call "HoloPy_Find_Features.vi"("imageNumber"=w354, "Threshold"=w366, "Refnum in"=w365) -> ("error out"=w351:errorcluster, "FEATURES(µm)"=w352:sgl[][])  [unwired: 6 in, 1 out]
                n148 = case shown="True" w359 {
                  tunnel: w352 -> [w380 w393]
                  tunnel: [w375 w381] -> w358
                  tunnel: w354 -> [_ w389]
                  tunnel: w357 -> [_ w390]
                  frame True {
                    n149 = Array Size(array=w380) -> (size(s)=w379:i32[])
                    n150 = Index Array(array=w379) -> (element=w378:i32)  [unwired: 1 in]
                    n151 = Number To Decimal String(number=w378) -> (decimal integer string=w376:string)  [unwired: 1 in]
                    n152 = Concatenate Strings(w376, " features found.") -> (w375:string)
                  }
                  frame False {
                    n153 = Array Size(array=w393) -> (size(s)=w392:i32[])
                    n154 = Number To Decimal String(number=w390) -> (decimal integer string=w385:string)  [unwired: 1 in]
                    n155 = Number To Decimal String(number=w389) -> (decimal integer string=w387:string)  [unwired: 1 in]
                    n156 = Index Array(array=w392) -> (element=w391:i32)  [unwired: 1 in]
                    n157 = Number To Decimal String(number=w391) -> (decimal integer string=w383:string)  [unwired: 1 in]
                    n158 = Concatenate Strings("Holo n°", w387, "/", w385, ". " ("string"), w383, " features found.") -> (w381:string)
                  }
                }
                n159 = Bundle By Name(cluster=w363, "FEATURES(µm)"=w352, "Display"=w353, "Status"=w358) -> (w362:T11)
              }
              frame "Display" {
                n160 = Unbundle By Name(w405) -> ("PythonSession"=w407:refnum<k35>, "FEATURES(µm)"=w403:sgl[][])
                n161 = Variant To Data(error in=w402, type=T14 {"Display"=enum."HOLOGRAM", "Plane number"=0} ("output cluster"), Variant=w401) -> (data=w399:T14, error out=w397:errorcluster)
                n162 = Unbundle(w399) -> ("Display"=w396:T7, "Plane number"=w398:u16)
                n163 = Select(t=T7."HOLOGRAM", s=w397, f=w396) -> (s? t:f=w395:T7)
                n164 = case shown="\"XY PLANE NUMBER....\"" w395 {
                  tunnel: w407 -> [w428 w435 w455 w474 w494 w514 w534 w554]
                  tunnel: [w427 w451 w471 w491 w511 w531 w551 w571] -> w406
                  tunnel: w404 -> [w426 w450 w470 w490 w510 w530 w550 w570]
                  tunnel: w403 -> [w413 w439 w459 w479 w499 w519 w539 w559]
                  tunnel: w398 -> [_ w429 _ _ _ _ _ _]
                  frame "HOLOGRAM", Default {
                    n165 = call "HoloPy_get_hologram.vi"("Refnum in"=w428) -> ("error out"=w421:errorcluster, "HOLO_array"=w417:sgl[][])  [unwired: 8 in, 1 out]
                    n166 = local read "propagation"() -> (w425:T5)
                    n167 = local read "HoloParam"() -> (w422:T6)
                    n168 = Unbundle By Name(w422) -> ("pixel size"=w424:sgl, "objective magnification"=w423:sgl)
                    n169 = Unbundle By Name(w425) -> ("step"=w412:dbl)
                    n170 = Divide(x=w424, y=w423) -> (x/y=w411:sgl)
                    n171 = call "scaleFeaturesPositions_um_pix.vi"("error in (no error)"=w421, "dXY"=w411, "dZ"=w412, "FEATURES(µm)"=w413) -> ("error out"=w420:errorcluster, "Features(pix)"=w416:sgl[][])  [unwired: 6 in]
                    n172 = Bundle(cluster=T15 {"HOLO_array"=[], "FEATURES(µm)"=[], "Features(pix)"=[], "planeToDisplayFeatures"=enum."XY", "label"=""} ("output cluster"), "HOLO_array"=w417, "FEATURES(µm)"=w413, "Features(pix)"=w416, "planeToDisplayFeatures"=enum16{"XY", "XZ", "YZ"}."XY", "label"="Hologram" ("command")) -> (w415:T15)
                    n173 = Bundle By Name(cluster=cluster{"command":string, "data":variant} {"command"="updateDisplay", "data"=variant} ("element"), "data"=w415) -> (w418:cluster{"command":string, "data":variant})
                    n174 = Enqueue Element(queue=w426, element=w418, error in (no error)=w420) -> (error out=w427:errorcluster)  [unwired: 1 in, 2 out]
                  }
                  frame "XY PLANE NUMBER...." {
                    n175 = call "HoloPy_get_reconstruction_plane.vi"("plane number"=w429, "Refnum in"=w435) -> ("error out"=w434:errorcluster, "HOLO_array"=w433:sgl[][])  [unwired: 7 in, 1 out]
                    n176 = local read "propagation"() -> (w449:T5)
                    n177 = local read "HoloParam"() -> (w446:T6)
                    n178 = Unbundle By Name(w446) -> ("pixel size"=w448:sgl, "objective magnification"=w447:sgl)
                    n179 = Number To Decimal String(number=w429) -> (decimal integer string=w432:string)  [unwired: 1 in]
                    n180 = Unbundle By Name(w449) -> ("step"=w438:dbl)
                    n181 = Concatenate Strings("Hologram plane number " ("Label.Text"), w432) -> (w430:string)
                    n182 = Divide(x=w448, y=w447) -> (x/y=w437:sgl)
                    n183 = call "scaleFeaturesPositions_um_pix.vi"("error in (no error)"=w434, "dXY"=w437, "dZ"=w438, "FEATURES(µm)"=w439) -> ("error out"=w445:errorcluster, "Features(pix)"=w442:sgl[][])  [unwired: 6 in]
                    n184 = Bundle(cluster=T15 {"HOLO_array"=[], "FEATURES(µm)"=[], "Features(pix)"=[], "planeToDisplayFeatures"=enum."XY", "label"=""} ("output cluster"), "HOLO_array"=w433, "FEATURES(µm)"=w439, "Features(pix)"=w442, "planeToDisplayFeatures"=enum16{"XY", "XZ", "YZ"}."XY", "label"=w430) -> (w441:T15)
                    n185 = Bundle By Name(cluster=cluster{"command":string, "data":variant} {"command"="updateDisplay", "data"=variant} ("element"), "data"=w441) -> (w443:cluster{"command":string, "data":variant})
                    n186 = Enqueue Element(queue=w450, element=w443, error in (no error)=w445) -> (error out=w451:errorcluster)  [unwired: 1 in, 2 out]
                  }
                  frame "XY MAX PLANE" {
                    n187 = call "HoloPy_max_XY_planes_from_volume.vi"("Refnum in"=w455) -> ("error out"=w453:errorcluster, "XY Plane"=w454:sgl[][])  [unwired: 8 in, 1 out]
                    n188 = local read "propagation"() -> (w469:T5)
                    n189 = local read "HoloParam"() -> (w466:T6)
                    n190 = Unbundle By Name(w466) -> ("pixel size"=w468:sgl, "objective magnification"=w467:sgl)
                    n191 = Unbundle By Name(w469) -> ("step"=w458:dbl)
                    n192 = Divide(x=w468, y=w467) -> (x/y=w457:sgl)
                    n193 = call "scaleFeaturesPositions_um_pix.vi"("error in (no error)"=w453, "dXY"=w457, "dZ"=w458, "FEATURES(µm)"=w459) -> ("error out"=w465:errorcluster, "Features(pix)"=w462:sgl[][])  [unwired: 6 in]
                    n194 = Bundle(cluster=T15 {"HOLO_array"=[], "FEATURES(µm)"=[], "Features(pix)"=[], "planeToDisplayFeatures"=enum."XY", "label"=""} ("output cluster"), "HOLO_array"=w454, "FEATURES(µm)"=w459, "Features(pix)"=w462, "planeToDisplayFeatures"=enum16{"XY", "XZ", "YZ"}."XY", "label"="XY max focus plane projection" ("Label.Text")) -> (w461:T15)
                    n195 = Bundle By Name(cluster=cluster{"command":string, "data":variant} {"command"="updateDisplay", "data"=variant} ("element"), "data"=w461) -> (w463:cluster{"command":string, "data":variant})
                    n196 = Enqueue Element(queue=w470, element=w463, error in (no error)=w465) -> (error out=w471:errorcluster)  [unwired: 1 in, 2 out]
                  }
                  frame "XY SUM PLANE" {
                    n197 = call "HoloPy_sum_XY_planes_from_volume.vi"("Refnum in"=w474) -> ("error out"=w472:errorcluster, "XY Plane"=w473:sgl[][])  [unwired: 8 in, 1 out]
                    n198 = local read "propagation"() -> (w489:T5)
                    n199 = local read "HoloParam"() -> (w486:T6)
                    n200 = Unbundle By Name(w486) -> ("pixel size"=w488:sgl, "objective magnification"=w487:sgl)
                    n201 = Unbundle By Name(w489) -> ("step"=w478:dbl)
                    n202 = Divide(x=w488, y=w487) -> (x/y=w477:sgl)
                    n203 = call "scaleFeaturesPositions_um_pix.vi"("error in (no error)"=w472, "dXY"=w477, "dZ"=w478, "FEATURES(µm)"=w479) -> ("error out"=w485:errorcluster, "Features(pix)"=w482:sgl[][])  [unwired: 6 in]
                    n204 = Bundle(cluster=T15 {"HOLO_array"=[], "FEATURES(µm)"=[], "Features(pix)"=[], "planeToDisplayFeatures"=enum."XY", "label"=""} ("output cluster"), "HOLO_array"=w473, "FEATURES(µm)"=w479, "Features(pix)"=w482, "planeToDisplayFeatures"=enum16{"XY", "XZ", "YZ"}."XY", "label"="XY sum focus plane projection" ("Label.Text")) -> (w481:T15)
                    n205 = Bundle By Name(cluster=cluster{"command":string, "data":variant} {"command"="updateDisplay", "data"=variant} ("element"), "data"=w481) -> (w483:cluster{"command":string, "data":variant})
                    n206 = Enqueue Element(queue=w490, element=w483, error in (no error)=w485) -> (error out=w491:errorcluster)  [unwired: 1 in, 2 out]
                  }
                  frame "XZ MAX PLANE" {
                    n207 = call "HoloPy_max_XZ_planes_from_volume.vi"("Refnum in"=w494) -> ("error out"=w492:errorcluster, "XZ Plane"=w493:sgl[][])  [unwired: 8 in, 1 out]
                    n208 = local read "propagation"() -> (w509:T5)
                    n209 = local read "HoloParam"() -> (w506:T6)
                    n210 = Unbundle By Name(w506) -> ("pixel size"=w508:sgl, "objective magnification"=w507:sgl)
                    n211 = Unbundle By Name(w509) -> ("step"=w498:dbl)
                    n212 = Divide(x=w508, y=w507) -> (x/y=w497:sgl)
                    n213 = call "scaleFeaturesPositions_um_pix.vi"("error in (no error)"=w492, "dXY"=w497, "dZ"=w498, "FEATURES(µm)"=w499) -> ("error out"=w505:errorcluster, "Features(pix)"=w502:sgl[][])  [unwired: 6 in]
                    n214 = Bundle(cluster=T15 {"HOLO_array"=[], "FEATURES(µm)"=[], "Features(pix)"=[], "planeToDisplayFeatures"=enum."XY", "label"=""} ("output cluster"), "HOLO_array"=w493, "FEATURES(µm)"=w499, "Features(pix)"=w502, "planeToDisplayFeatures"=enum16{"XY", "XZ", "YZ"}."XZ", "label"="XZ  max focus plane projection" ("Label.Text")) -> (w501:T15)
                    n215 = Bundle By Name(cluster=cluster{"command":string, "data":variant} {"command"="updateDisplay", "data"=variant} ("element"), "data"=w501) -> (w503:cluster{"command":string, "data":variant})
                    n216 = Enqueue Element(queue=w510, element=w503, error in (no error)=w505) -> (error out=w511:errorcluster)  [unwired: 1 in, 2 out]
                  }
                  frame "XZ SUM PLANE" {
                    n217 = call "HoloPy_sum_XZ_planes_from_volume.vi"("Refnum in"=w514) -> ("error out"=w512:errorcluster, "XZ Plane"=w513:sgl[][])  [unwired: 8 in, 1 out]
                    n218 = local read "propagation"() -> (w529:T5)
                    n219 = local read "HoloParam"() -> (w526:T6)
                    n220 = Unbundle By Name(w526) -> ("pixel size"=w528:sgl, "objective magnification"=w527:sgl)
                    n221 = Unbundle By Name(w529) -> ("step"=w518:dbl)
                    n222 = Divide(x=w528, y=w527) -> (x/y=w517:sgl)
                    n223 = call "scaleFeaturesPositions_um_pix.vi"("error in (no error)"=w512, "dXY"=w517, "dZ"=w518, "FEATURES(µm)"=w519) -> ("error out"=w525:errorcluster, "Features(pix)"=w522:sgl[][])  [unwired: 6 in]
                    n224 = Bundle(cluster=T15 {"HOLO_array"=[], "FEATURES(µm)"=[], "Features(pix)"=[], "planeToDisplayFeatures"=enum."XY", "label"=""} ("output cluster"), "HOLO_array"=w513, "FEATURES(µm)"=w519, "Features(pix)"=w522, "planeToDisplayFeatures"=enum16{"XY", "XZ", "YZ"}."XZ", "label"="XZ  sum focus plane projection" ("Label.Text")) -> (w521:T15)
                    n225 = Bundle By Name(cluster=cluster{"command":string, "data":variant} {"command"="updateDisplay", "data"=variant} ("element"), "data"=w521) -> (w523:cluster{"command":string, "data":variant})
                    n226 = Enqueue Element(queue=w530, element=w523, error in (no error)=w525) -> (error out=w531:errorcluster)  [unwired: 1 in, 2 out]
                  }
                  frame "YZ MAX PLANE" {
                    n227 = call "HoloPy_max_YZ_planes_from_volume.vi"("Refnum in"=w534) -> ("error out"=w532:errorcluster, "YZ Plane"=w533:sgl[][])  [unwired: 8 in, 1 out]
                    n228 = local read "propagation"() -> (w549:T5)
                    n229 = local read "HoloParam"() -> (w546:T6)
                    n230 = Unbundle By Name(w546) -> ("pixel size"=w548:sgl, "objective magnification"=w547:sgl)
                    n231 = Unbundle By Name(w549) -> ("step"=w538:dbl)
                    n232 = Divide(x=w548, y=w547) -> (x/y=w537:sgl)
                    n233 = call "scaleFeaturesPositions_um_pix.vi"("error in (no error)"=w532, "dXY"=w537, "dZ"=w538, "FEATURES(µm)"=w539) -> ("error out"=w545:errorcluster, "Features(pix)"=w542:sgl[][])  [unwired: 6 in]
                    n234 = Bundle(cluster=T15 {"HOLO_array"=[], "FEATURES(µm)"=[], "Features(pix)"=[], "planeToDisplayFeatures"=enum."XY", "label"=""} ("output cluster"), "HOLO_array"=w533, "FEATURES(µm)"=w539, "Features(pix)"=w542, "planeToDisplayFeatures"=enum16{"XY", "XZ", "YZ"}."YZ", "label"="YZ max focus plane projection" ("Label.Text")) -> (w541:T15)
                    n235 = Bundle By Name(cluster=cluster{"command":string, "data":variant} {"command"="updateDisplay", "data"=variant} ("element"), "data"=w541) -> (w543:cluster{"command":string, "data":variant})
                    n236 = Enqueue Element(queue=w550, element=w543, error in (no error)=w545) -> (error out=w551:errorcluster)  [unwired: 1 in, 2 out]
                  }
                  frame "YZ SUM PLANE" {
                    n237 = call "HoloPy_sum_YZ_planes_from_volume.vi"("Refnum in"=w554) -> ("error out"=w552:errorcluster, "YZ Plane"=w553:sgl[][])  [unwired: 8 in, 1 out]
                    n238 = local read "propagation"() -> (w569:T5)
                    n239 = local read "HoloParam"() -> (w566:T6)
                    n240 = Unbundle By Name(w566) -> ("pixel size"=w568:sgl, "objective magnification"=w567:sgl)
                    n241 = Unbundle By Name(w569) -> ("step"=w558:dbl)
                    n242 = Divide(x=w568, y=w567) -> (x/y=w557:sgl)
                    n243 = call "scaleFeaturesPositions_um_pix.vi"("error in (no error)"=w552, "dXY"=w557, "dZ"=w558, "FEATURES(µm)"=w559) -> ("error out"=w565:errorcluster, "Features(pix)"=w562:sgl[][])  [unwired: 6 in]
                    n244 = Bundle(cluster=T15 {"HOLO_array"=[], "FEATURES(µm)"=[], "Features(pix)"=[], "planeToDisplayFeatures"=enum."XY", "label"=""} ("output cluster"), "HOLO_array"=w553, "FEATURES(µm)"=w559, "Features(pix)"=w562, "planeToDisplayFeatures"=enum16{"XY", "XZ", "YZ"}."YZ", "label"="YZ sum focus plane projection" ("Label.Text")) -> (w561:T15)
                    n245 = Bundle By Name(cluster=cluster{"command":string, "data":variant} {"command"="updateDisplay", "data"=variant} ("element"), "data"=w561) -> (w563:cluster{"command":string, "data":variant})
                    n246 = Enqueue Element(queue=w570, element=w563, error in (no error)=w565) -> (error out=w571:errorcluster)  [unwired: 1 in, 2 out]
                  }
                }
              }
              frame "displayHolo" {
                n247 = Unbundle By Name(w579) -> ("PythonSession"=w573:refnum<k35>)
                n248 = call "HoloPy_get_hologram.vi"("error in (no error)"=w575, "Refnum in"=w573) -> ("error out"=w574:errorcluster)  [unwired: 7 in, 2 out]
                n249 = Bundle By Name(cluster=w579, "LabelPicture"="Hologram" ("Label.Text"), "planeToDisplayFeatures"=enum16{"XY", "XZ", "YZ"}."XY", "Display"=TRUE) -> (w578:T11)
              }
              frame "displaySubVolume" {
                n250 = Unbundle By Name(w593) -> ("PythonSession"=w588:refnum<k35>)
                n251 = Variant To Data(error in=w587, type=T16 {"X"=0, "Y"=0, "Z"=0, "XYsize"=0, "ZSize"=0} ("param"), Variant=w586) -> (data=w584:T16, error out=w583:errorcluster)
                n252 = call "HoloPy_subvolume_3planes.vi"("error in (no error)"=w583, "param"=w584, "Refnum in"=w588) -> ("error out"=w589:errorcluster)  [unwired: 6 in, 2 out]
                n253 = Bundle By Name(cluster=w593, "LabelPicture"="sub volume 3 planes" ("Label.Text"), "planeToDisplayFeatures"=enum16{"XY", "XZ", "YZ"}."XY", "Display"=TRUE) -> (w592:T11)
              }
              frame "displayHolo_plane" {
                w600 = u16 0 ("Plane number")
                (unwired) "Hologram plane" ("Label.Text")
                n254 = Variant To Data(error in=w610, type=w600, Variant=w609) -> (data=w606:u16, error out=w608:errorcluster)
                n255 = Unbundle By Name(w605) -> ("PythonSession"=w607:refnum<k35>)
                n256 = call "HoloPy_get_reconstruction_plane.vi"("error in (no error)"=w608, "plane number"=w606, "Refnum in"=w607) -> ("error out"=w598:errorcluster)  [unwired: 6 in, 2 out]
                n257 = Number To Decimal String(number=w600) -> (decimal integer string=w599:string)  [unwired: 1 in]
                n258 = Concatenate Strings("Hologram plane number " ("Label.Text"), w599) -> (w601:string)
                n259 = Bundle By Name(cluster=w605, "LabelPicture"=w601, "planeToDisplayFeatures"=enum16{"XY", "XZ", "YZ"}."XY", "Display"=TRUE) -> (w604:T11)
              }
              frame "displayBin_plane" {
                w619 = u16 0 ("Plane number")
                n260 = Variant To Data(error in=w626, type=w619, Variant=w625) -> (data=w616:u16, error out=w617:errorcluster)
                n261 = Unbundle By Name(w624) -> ("PythonSession"=w615:refnum<k35>)
                n262 = call "HoloPy_get_binarised_plane.vi"("error in (no error)"=w617, "plane number"=w616, "Refnum in"=w615) -> ("error out"=w614:errorcluster)  [unwired: 6 in, 2 out]
                n263 = Number To Decimal String(number=w619) -> (decimal integer string=w618:string)  [unwired: 1 in]
                n264 = Concatenate Strings("Hologram bin plane number " ("Label.Text"), w618) -> (w620:string)
                n265 = Bundle By Name(cluster=w624, "LabelPicture"=w620, "planeToDisplayFeatures"=enum16{"XY", "XZ", "YZ"}."XY", "Display"=TRUE) -> (w623:T11)
              }
              frame "TEST SUM BIN PLANE" {
                n266 = Unbundle By Name(w636) -> ("PythonSession"=w631:refnum<k35>)
                n267 = call "HoloPy_get_sum_bin_planes.vi"("error in (no error)"=w630, "Refnum in"=w631) -> ("error out"=w633:errorcluster, "XY Plane"=w632:i32[][])  [unwired: 7 in, 1 out]
                n268 = To Single Precision Float(number=w632) -> ()  [unwired: 1 out]
                n269 = Bundle By Name(cluster=w636, "LabelPicture"="Sum thresholded planes" ("Label.Text"), "Display"=TRUE) -> (w635:T11)
              }
              frame "savePosition" {
                n270 = Variant To Data(error in=w647, type=path "" ("Holograms directory"), Variant=w646) -> (data=w641:path, error out=w644:errorcluster)
                n271 = Unbundle By Name(w640) -> ("PythonSession"=w642:refnum<k35>, "FEATURES(µm)"=w639:sgl[][])
                n272 = call "HoloPy_save_Features_csv.vi"("error in (no error)"=w644, "path csv file"=w641, "Array"=w639, "Refnum in"=w642) -> ("error out"=w643:errorcluster)  [unwired: 6 in, 1 out]
              }
            }
            n273 = Unbundle By Name(w90) -> ("State"=w89:T10)
            n274 = call "displayMessageSender.vi"("error in (no error)"=w92, "DatasIN"=w90, "QueueMsgIN"=w94) -> ("error out"=w93:errorcluster, "DatasOUT"=w91:T11)  [unwired: 6 in, 1 out]
            n275 = global write "globState.vi" "State"(w89) -> ()
          }
          frame Error {
            n276 = flat-sequence {
              tunnel: w654 -> [w656]
              tunnel: w653 -> [w657]
              tunnel: [w657] -> w652
              tunnel: w652 -> [w659]
              frame #0 {
                n277 = Flush Queue(queue=w656) -> (queue out=w655:refnum<queue>)  [unwired: 1 in, 2 out]
                n278 = Enqueue Element(queue=w655, element=cluster{"command":string, "data":variant} {"command"="closePythonSession", "data"=variant}) -> ()  [unwired: 2 in, 3 out]
              }
              frame #1 {
                n279 = call <vilib>:"Simple Error Handler.vi"("error in (no error)"=w659) -> ()  [unwired: 4 in, 5 out]
              }
            }
          }
        }
      }
      n280 = while {
        tunnel: w80 -> [w663]
        tunnel: w79 -> [w662]
        tunnel: [w661] -> w78
        tunnel: w75 -> [w660]
        stop <- w664 stop-if-true
        # "USER EVENT"
        n281 = event shown="[4] \"testMode\": Value Change" {
          selector: w662 -> [_ _ _ _ _ _ _ _ _ _ _]
          dyn-events: _ -> [_ _ _ _ _ _ _ _ _ _ _]
          timeout: _ -> [_ _ _ _ _ _ _ _ _ _ _]
          tunnel: [FALSE FALSE TRUE _ _ _ _ _ _ _ _] -> w664
          tunnel: w663 -> [w669 w677 _ w687 w702 w712 w719 w727 w736 w738 w746]
          tunnel: [w665 w676 _ _ _ _ _ _ _ _ _] -> w661
          tunnel: w660 -> [w667 w671 _ _ _ _ _ _ _ _ _]
          event "EXIT": Value Change {
            w668 = cluster{"command":string, "data":variant} {"command"="EXIT", "data"=variant} ("element")
            n282 = event-data() -> ()  [unwired: 1 in, 1 out]
            n283 = Enqueue Element(queue=w669, element=w668) -> (error out=w666:errorcluster)  [unwired: 2 in, 2 out]
            n284 = Enqueue Element(queue=w667, element=w668, error in (no error)=w666) -> (error out=w665:errorcluster)  [unwired: 1 in, 2 out]
          }
          event Panel Close? {
            n285 = event-data() -> ()  [unwired: 1 in, 4 out]
            n286 = Two Button Dialog(message="EXIT APPLICATION?", 2:"YES" ("T button name (\"OK\")")) -> (T button?=w673:bool)  [unwired: 1 in]
            n287 = case shown="True" w673 {
              tunnel: w677 -> [_ w684]
              tunnel: [errorcluster {"status"=FALSE, "code"=0, "source"=""} ("error out") w680] -> w676
              tunnel: w671 -> [_ w682]
              frame False {
              }
              frame True {
                w681 = cluster{"command":string, "data":variant} {"command"="EXIT", "data"=variant} ("element")
                n288 = Enqueue Element(queue=w684, element=w681) -> (error out=w683:errorcluster)  [unwired: 2 in, 2 out]
                n289 = Enqueue Element(queue=w682, element=w681, error in (no error)=w683) -> (error out=w680:errorcluster)  [unwired: 1 in, 2 out]
              }
            }
            n290 = event-data("Discard?"=TRUE) -> ()  [unwired: 1 in, 1 out]
          }
          event User Event {
            n291 = event-data() -> ()  [unwired: 1 in, 5 out]
          }
          event "propagation", "HoloDir", "Remove mean Hologram": Value Change {
            n292 = event-data() -> ()  [unwired: 1 in, 1 out]
            n293 = global read "globState.vi" "State"() -> (w686:T10)
            n294 = case shown="\"TEST WAIT\"" w686 {
              tunnel: w687 -> [_ w688]
              frame "WAIT", Default {
              }
              frame "TEST WAIT" {
                n295 = local read "Remove mean Hologram"() -> (w689:bool)
                n296 = Select(t=string[] ["startTest", "allocate", "openHolo", "Display", "get holo path list", "computeMeanHolo", "removeMeanHolo", "Display", "reconstructAndFocus", "computeThreshold", "findFeatures", "test finished", "Display"], s=w689, f=string[] ["startTest", "allocate", "openHolo", "Display", "reconstructAndFocus", "computeThreshold", "findFeatures", "test finished", "Display"]) -> (s? t:f=w690:string[])
                n297 = for {
                  tunnel: w688 -> [w697]
                  tunnel: w690 -> [w695] mode=indexing
                  tunnel: [w693] -> _ mode=indexing
                  n298 = Bundle By Name(cluster=cluster{"command":string, "data":variant} {"command"="", "data"=variant} ("element"), "command"=w695) -> (w694:cluster{"command":string, "data":variant})
                  n299 = Enqueue Element(queue=w697, element=w694) -> (error out=w693:errorcluster)  [unwired: 2 in, 2 out]
                }
              }
            }
          }
          event "testMode": Value Change {
            n300 = event-data() -> ()  [unwired: 1 in, 6 out]
            n301 = Select(t=string[] ["openPythonSession", "startTest", "allocate", "openHolo", "Display", "get holo path list", "computeMeanHolo", "removeMeanHolo", "Display", "reconstructAndFocus", "computeThreshold", "findFeatures", "test finished", "Display"], s="Remove mean Hologram", f=string[] ["openPythonSession", "startTest", "allocate", "openHolo", "Display", "reconstructAndFocus", "computeThreshold", "findFeatures", "test finished", "Display"]) -> (s? t:f=w699:string[])
            n302 = for {
              tunnel: w702 -> [w707]
              tunnel: w699 -> [w705] mode=indexing
              tunnel: [w703] -> _ mode=indexing
              n303 = Bundle By Name(cluster=cluster{"command":string, "data":variant} {"command"="", "data"=variant} ("element"), "command"=w705) -> (w704:cluster{"command":string, "data":variant})
              n304 = Enqueue Element(queue=w707, element=w704) -> (error out=w703:errorcluster)  [unwired: 2 in, 2 out]
            }
          }
          event "BATCH": Value Change {
            n305 = event-data() -> ()  [unwired: 1 in, 6 out]
            n306 = local read "Remove mean Hologram"() -> (w710:bool)
            n307 = Select(t=string[] ["openPythonSession", "statusBatch", "allocate", "get holo path list", "computeMeanHolo", "start batch"], s=w710, f=string[] ["openPythonSession", "statusBatch", "allocate", "get holo path list", "start batch"]) -> (s? t:f=w711:string[])
            n308 = for {
              tunnel: w712 -> [w717]
              tunnel: w711 -> [w715] mode=indexing
              tunnel: [w713] -> _ mode=indexing
              n309 = Bundle By Name(cluster=cluster{"command":string, "data":variant} {"command"="", "data"=variant} ("element"), "command"=w715) -> (w714:cluster{"command":string, "data":variant})
              n310 = Enqueue Element(queue=w717, element=w714) -> (error out=w713:errorcluster)  [unwired: 2 in, 2 out]
            }
          }
          event "Fourier BP filter (pix)", "Focus": Value Change {
            n311 = event-data() -> ()  [unwired: 1 in, 1 out]
            n312 = global read "globState.vi" "State"() -> (w718:T10)
            n313 = case shown="\"TEST WAIT\"" w718 {
              tunnel: w719 -> [_ w721]
              frame "WAIT", Default {
              }
              frame "TEST WAIT" {
                n314 = for {
                  tunnel: w721 -> [w726]
                  tunnel: string[] ["setParam", "reconstructAndFocus", "computeThreshold", "findFeatures", "test finished", "Display"] -> [w724] mode=indexing
                  tunnel: [w722] -> _ mode=indexing
                  n315 = Bundle By Name(cluster=cluster{"command":string, "data":variant} {"command"="", "data"=variant} ("element"), "command"=w724) -> (w723:cluster{"command":string, "data":variant})
                  n316 = Enqueue Element(queue=w726, element=w723) -> (error out=w722:errorcluster)  [unwired: 2 in, 2 out]
                }
              }
            }
          }
          event "exitTestMode": Value Change {
            n317 = event-data() -> ()  [unwired: 1 in, 6 out]
            n318 = Flush Queue(queue=w727) -> (queue out=w729:refnum<queue>)  [unwired: 1 in, 2 out]
            n319 = for {
              tunnel: w729 -> [w734]
              tunnel: string[] ["stopTest", "closePythonSession"] -> [w732] mode=indexing
              tunnel: [w730] -> _ mode=indexing
              n320 = Bundle By Name(cluster=cluster{"command":string, "data":variant} {"command"="", "data"=variant} ("element"), "command"=w732) -> (w731:cluster{"command":string, "data":variant})
              n321 = Enqueue Element(queue=w734, element=w731) -> (error out=w730:errorcluster)  [unwired: 2 in, 2 out]
            }
          }
          event "CANCEL_BATCH": Value Change {
            n322 = event-data() -> ()  [unwired: 1 in, 6 out]
            n323 = Enqueue Element At Opposite End(queue=w736, element=cluster{"command":string, "data":variant} {"command"="cancelBatch", "data"=variant}) -> ()  [unwired: 2 in, 3 out]
          }
          event "Display", "Plane number": Value Change {
            n324 = event-data() -> ()  [unwired: 1 in, 6 out]
            n325 = global read "globState.vi" "State"() -> (w737:T10)
            n326 = case shown="\"TEST WAIT\"" w737 {
              tunnel: w738 -> [_ _ w744 _ _]
              frame "SESSION CLOSED", Default {
              }
              frame "WAIT" {
              }
              frame "TEST WAIT" {
                n327 = Bundle("Display"="Display", "Plane number"="Plane number") -> (w741:T14)  [unwired: 1 in]
                n328 = Bundle By Name(cluster=cluster{"command":string, "data":variant} {"command"="Display", "data"=variant} ("element"), "data"=w741) -> (w740:cluster{"command":string, "data":variant})
                n329 = Enqueue Element(queue=w744, element=w740) -> ()  [unwired: 2 in, 3 out]
              }
              frame "TEST IN PROGESS" {
              }
              frame "BATCH IN PROGRESS" {
              }
            }
          }
          event Key Down {
            n330 = event-data() -> ("VKey"=w747:T17)  [unwired: 1 in, 8 out]
            n331 = local read "propagation"() -> (w745:T5)
            n332 = case shown="\"PageDown\"" w747 {
              tunnel: w746 -> [_ w748 w762]
              tunnel: w745 -> [_ _ w761]
              frame "ASCII", Default {
              }
              frame "PageDown" {
                n333 = global read "globState.vi" "State"() -> (w749:T10)
                n334 = case shown="\"TEST WAIT\"" w749 {
                  tunnel: w748 -> [_ _ w753 _ _]
                  frame "SESSION CLOSED", Default {
                  }
                  frame "WAIT" {
                  }
                  frame "TEST WAIT" {
                    n335 = local read "Plane number"() -> (w752:u16)
                    n336 = Decrement(x=w752) -> (x-1=w751:u16)
                    n337 = Greater Than 0?(x=w751) -> (x > 0?=w750:bool)
                    n338 = case shown="True" w750 {
                      tunnel: w753 -> [_ w759]
                      tunnel: w751 -> [_ w755]
                      frame False {
                      }
                      frame True {
                        n339 = local read "Display"() -> (w754:T7)
                        n340 = Bundle("Display"=w754, w755) -> (w758:T18)  [unwired: 1 in]
                        n341 = Bundle By Name(cluster=cluster{"command":string, "data":variant} {"command"="Display", "data"=variant} ("element"), "data"=w758) -> (w757:cluster{"command":string, "data":variant})
                        n342 = local write "Plane number"(w755) -> ()
                        n343 = Enqueue Element(queue=w759, element=w757) -> ()  [unwired: 2 in, 3 out]
                      }
                    }
                  }
                  frame "TEST IN PROGESS" {
                  }
                  frame "BATCH IN PROGRESS" {
                  }
                }
              }
              frame "PageUp" {
                n344 = Unbundle By Name(w761) -> ("number of planes"=w760:i32)
                n345 = global read "globState.vi" "State"() -> (w763:T10)
                n346 = case shown="\"TEST WAIT\"" w763 {
                  tunnel: w762 -> [_ _ w768 _ _]
                  tunnel: w760 -> [_ _ w764 _ _]
                  frame "SESSION CLOSED", Default {
                  }
                  frame "WAIT" {
                  }
                  frame "TEST WAIT" {
                    n347 = local read "Plane number"() -> (w767:u16)
                    n348 = Increment(x=w767) -> (x+1=w765:u16)
                    n349 = Less?(x=w765, y=w764) -> (x < y?=w766:bool)
                    n350 = case shown="True" w766 {
                      tunnel: w768 -> [_ w774]
                      tunnel: w765 -> [_ w770]
                      frame False {
                      }
                      frame True {
                        n351 = local read "Display"() -> (w769:T7)
                        n352 = Bundle("Display"=w769, w770) -> (w773:T18)  [unwired: 1 in]
                        n353 = Bundle By Name(cluster=cluster{"command":string, "data":variant} {"command"="Display", "data"=variant} ("element"), "data"=w773) -> (w772:cluster{"command":string, "data":variant})
                        n354 = local write "Plane number"(w770) -> ()
                        n355 = Enqueue Element(queue=w774, element=w772) -> ()  [unwired: 2 in, 3 out]
                      }
                    }
                  }
                  frame "TEST IN PROGESS" {
                  }
                  frame "BATCH IN PROGRESS" {
                  }
                }
              }
            }
          }
        }
      }
      n356 = while {
        tunnel: w75 -> [w783]
        tunnel: w77 -> [w777]
        tunnel: [w776] -> w74
        tunnel: w72 -> [w775]
        stop <- w778 stop-if-true
        # "DISPLAY AND SAVE"
        n357 = Dequeue Element(queue=w783) -> (element=w781:cluster{"command":string, "data":variant}, error out=w782:errorcluster)  [unwired: 2 in, 2 out]
        n358 = Unbundle(w781) -> ("command"=w780:string, "data"=w779:variant)
        n359 = case shown="\"updateStatus\"" w780 {
          tunnel: w782 -> [w784 w791 w799 w815 w833 w834]
          tunnel: w779 -> [_ w790 w798 w814 w832 _]
          tunnel: [FALSE FALSE FALSE FALSE FALSE TRUE] -> w778
          tunnel: w777 -> [_ _ _ _ _ w836]
          tunnel: [w784 w787 w796 w810 w830 w834] -> w776
          tunnel: w775 -> [_ _ w794 _ _ _]
          frame "", Default {
          }
          frame "updateStatus" {
            n360 = Variant To Data(error in=w791, type="" ("return value"), Variant=w790) -> (data=→"Status":string, error out=w787:errorcluster)
          }
          frame "updateBtnIHM" {
            n361 = Variant To Data(error in=w799, type=T10."SESSION CLOSED" ("State"), Variant=w798) -> (data=w793:T10, error out=w795:errorcluster)
            n362 = call "activateBtnIHM.vi"("error in (no error)"=w795, "State"=w793, "References"=w794) -> ("error out"=w796:errorcluster)  [unwired: 8 in]
          }
          frame "updateDisplay" {
            n363 = Variant To Data(error in=w815, type=T15 {"HOLO_array"=[], "FEATURES(µm)"=[], "Features(pix)"=[], "planeToDisplayFeatures"=enum."XY", "label"=""} ("output cluster"), Variant=w814) -> (data=w812:T15, error out=w801:errorcluster)
            n364 = Unbundle(w812) -> ("HOLO_array"=w806:sgl[][], "FEATURES(µm)"=w805:sgl[][], "Features(pix)"=w800:sgl[][], "planeToDisplayFeatures"=w802:enum16{"XY", "XZ", "YZ"}, "label"=w803:string)
            n365 = Not Equal?(x=w805, y=sgl[][] []) -> (x != y?=w808:bool)
            n366 = case shown="True" w808 {
              tunnel: w805 -> [_ w816]
              frame False {
              }
              frame True {
                w820 = 1000000.0
                n367 = Index Array(array=w816, index (col) #1=1 ("disabled index (col)"), index (col) #2=2 ("index (col)"), index (col) #3=3 ("index (col)")) -> (element #1=w821:sgl[], element #2=w822:sgl[], element #3=w823:sgl[])  [unwired: 3 in]
                n368 = Multiply(x=w822, y=w820) -> (x*y=w826:dbl[])
                n369 = Multiply(x=w821, y=w820) -> (x*y=w825:dbl[])
                n370 = Multiply(x=w823, y=w820) -> (x*y=w824:dbl[])
                n371 = call-poly <vilib>:"Plot Helper.vi"("z vector"=w824, "y vector"=w825, "x vector"=w826) -> ("3D Plot lvclass Array out"=→"3D Scatter":refnum<class "3D Plot Datatype.lvclass">[])  [unwired: 3 in, 5 out]
              }
            }
            n372 = control-ref of="2D Picture"() -> (w811:refnum<vi>)
            n373 = call "convert_float_array_to_U8_Picture.vi"("Pict Refnum"=w811, "error in (no error)"=w801, "planeToDisplayFeatures"=w802, "FEATURES (PIX)"=w800, "HOLO"=w806) -> ("error out"=w810:errorcluster, "new picture"=→"2D Picture":picture)  [unwired: 5 in]
            n374 = property on="2D Picture" class="Pict"("Caption.Text"=w803) -> ()  [unwired: 2 in, 2 out]
          }
          frame "updateLabelPicture" {
            n375 = Variant To Data(error in=w833, type="label" ("Label.Text"), Variant=w832) -> (data=w828:string, error out=w830:errorcluster)
            n376 = property on="2D Picture" class="Pict"("Caption.Text"=w828) -> ()  [unwired: 2 in, 2 out]
          }
          frame "EXIT" {
            n377 = Generate User Event(user event=w836, event data cluster=TRUE ("event data")) -> ()  [unwired: 2 in, 2 out]
          }
        }
      }
    }
    frame #2 {
      n378 = local read "Batch thresold"() -> (w850:T3)
      n379 = local read "PythonVer"() -> (w841:string)
      n380 = local read "Python/Environnement\npath"() -> (w842:path)
      n381 = local read "HoloPath"() -> (w843:path)
      n382 = local read "HoloDir"() -> (w844:path)
      n383 = local read "HoloParam"() -> (w845:T6)
      n384 = local read "Remove mean Hologram"() -> (w846:bool)
      n385 = local read "propagation"() -> (w847:T5)
      n386 = local read "Fourier BP filter (pix)"() -> (w848:T1)
      n387 = local read "Focus"() -> (w849:T4)
      n388 = local read "CCL parameters"() -> (w851:T2)
      n389 = Merge Errors(w854, w855, w856) -> (w853:errorcluster)
      n390 = Destroy User Event(user event=w857, error in=w853) -> (error out=w859:errorcluster)
      n391 = Unregister For Events(event registration refnum=w858, error in=w859) -> (error out=w838:errorcluster)
      n392 = Bundle("PythonVer"=w841, "Python/Environnement\npath"=w842, "HoloPath"=w843, "HoloDir"=w844, "HoloParam"=w845, "Remove mean Hologram"=w846, "propagation"=w847, "Fourier BP filter (pix)"=w848, "Focus"=w849, "Batch thresold"=w850, "CCL parameters"=w851) -> (w852:T19)  [unwired: 1 in]
      n393 = call "EcrireLireValeurParDefaut_HoloTrackPy_locate.vi"("Lecture/Ecriture"=enum32{"Lecture", "Ecriture"}."Ecriture", "ParamIN"=w852) -> ("error out"=w839:errorcluster)  [unwired: 6 in, 3 out]
      n394 = disable-structure shown="RUN_TIME_ENGINE==True" {
        disable-tunnel: w839 -> [_ _]
        disable-tunnel: w838 -> [_ _]
        frame condition #0 {
          n395 = Quit LabVIEW(quit? (T)=TRUE) -> ()
        }
        frame condition #1 (active) {
        }
      }
    }
  }
